vi "DSby4.vi"(11 "Element":cluster{"Older Data":u64, "Newer Data":u64}) -> (3 "Numeric":u32)   [LabVIEW 2020]
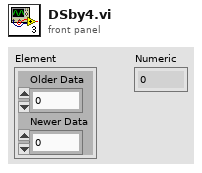
[diagram p1: front panel]
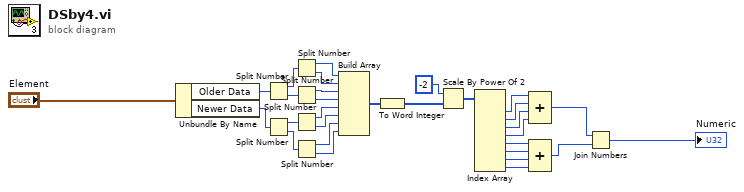
[diagram p0: block diagram]
diagram:
  n1 = Unbundle By Name("Element") -> ("Older Data"=w16:u64, "Newer Data"=w15:u64)
  n2 = Split Number(x=w16) -> (hi(x)=w17:u32, lo(x)=w14:u32)
  n3 = Split Number(x=w15) -> (hi(x)=w13:u32, lo(x)=w12:u32)
  n4 = Split Number(x=w17) -> (hi(x)=w18:u16, lo(x)=w11:u16)
  n5 = Split Number(x=w14) -> (hi(x)=w10:u16, lo(x)=w9:u16)
  n6 = Split Number(x=w13) -> (hi(x)=w8:u16, lo(x)=w7:u16)
  n7 = Split Number(x=w12) -> (hi(x)=w6:u16, lo(x)=w5:u16)
  n8 = Build Array(w18, w11, w10, w9, w8, w7, w6, w5) -> (w4:u16[])
  n9 = To Word Integer(number=w4) -> (16bit integer=w2:i16[])
  n10 = Scale By Power Of 2(n=i16 -2, x=w2) -> (x*2^n=w1:i16[])
  n11 = Index Array(array=w1) -> (element #1=w20:i16, element #2=w21:i16, element #3=w22:i16, element #4=w23:i16, element #5=w24:i16, element #6=w25:i16, element #7=w26:i16, element #8=w27:i16)  [unwired: 8 in]
  n12 = Compound Arithmetic op=ADD(w20, w21, w22, w23) -> (w28:i16)
  n13 = Compound Arithmetic op=ADD(w24, w25, w26, w27) -> (w29:i16)
  n14 = Join Numbers(hi=w28, lo=w29) -> ((hi.lo)=→"Numeric":u32)
